vi "Name to ref convert.vi"   [LabVIEW 2020]
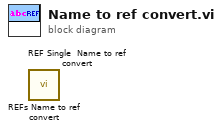
[diagram p0: block diagram]
diagram:
  n1 = call "REFs Name to ref convert.vi"() -> ()  [unwired: 11 in, 1 out]
  n2 = call "REF Single  Name to ref convert.vi"() -> ()  [unwired: 11 in, 1 out]
